vi "JKI_VI_Tester.vi"(11 "Args":string[](array[string])) -> (2 "Output":string, 3 "Exit Code":i32)   [LabVIEW 2020]
uses:
  <vilib>/addons/_JKI Toolkits/VI Tester/VI Tester API.llb/Run Tests (Path Array).vi
  <vilib>/addons/_JKI Toolkits/VI Tester/VI Tester API.llb/VI Tester API.lvlib
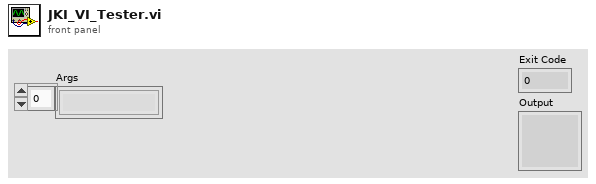
[diagram p1: front panel]
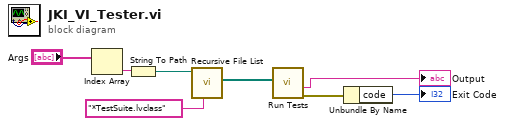
[diagram p0: block diagram]
diagram:
  n1 = Index Array(array="Args") -> (element=w4:string)  [unwired: 1 in]
  n2 = String To Path(string=w4) -> (path=w3:path)
  n3 = call <vilib>:"Recursive File List.vi"("pattern"="*TestSuite.lvclass", "Folder Path"=w3) -> ("All Files in Dir"=w1:path[])  [unwired: 5 in, 4 out]
  n4 = call-poly <vilib>:"Run Tests.vi"("Test Paths"=w1) -> ("error out"=w5:errorcluster, "test details"=→"Output":string)  [unwired: 8 in, 1 out]
  n5 = Unbundle By Name(w5) -> ("code"=→"Exit Code":i32)
